vi "SmoothWaveform.vi"(0 "Waveform":waveform(dbl)={"t0"=timestamp(3461330237.7970004 s since 1904-01-01), "dt"=9.000000000000001e-07, "Y"=[]}, 1 "Smoothing Strength":T1=enum."20") -> (2 "Filtered data":waveform(dbl)={"t0"=timestamp(3461330237.7970004 s since 1904-01-01), "dt"=9.000000000000001e-07, "Y"=[]})   [LabVIEW 2010]
uses:
  FilterStrength.ctl
  <vilib>/Analysis/3filter.llb/Filter Passband Type.ctl
  <vilib>/Analysis/3filter.llb/Butterworth Filter (DBL).vi
  <vilib>/Analysis/NI_AALBase.lvlib
panel:
  in  "Draw Graph":bool
  out "XY Graph":cluster{dbl[], dbl[]}[](graph)
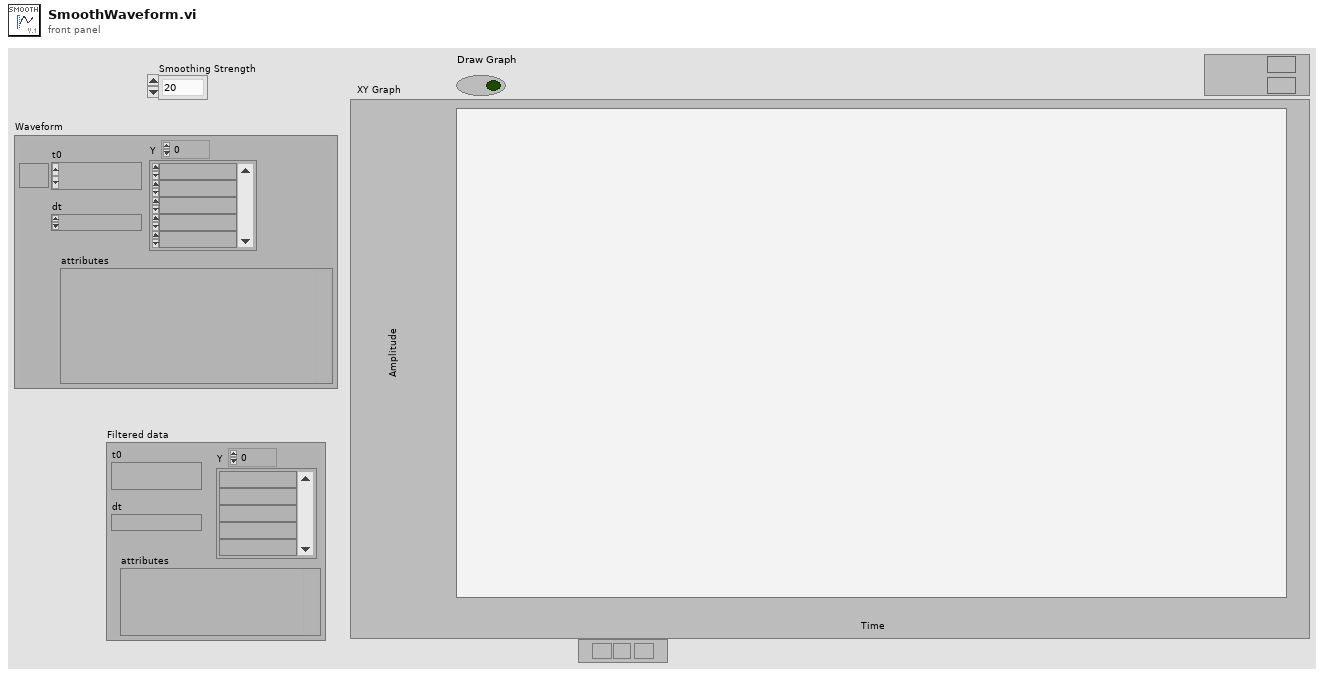
[diagram p1: front panel]
types:
  T1 = typedef "FilterStrength.ctl" = enum16{"Off", "10", "20", "50", "100", "200", "500", "1000"}
  T2 = typedef "NI_AALBase.lvlib/Filter Passband Type.ctl" = enum32{"Lowpass", "Highpass", "Bandpass", "Bandstop"}
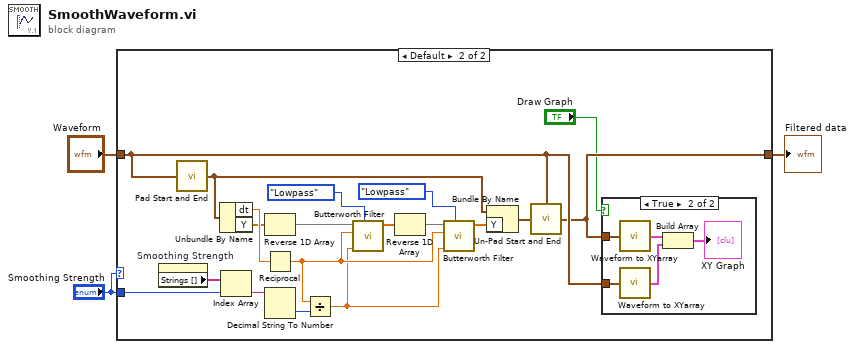
[diagram p0: block diagram]
diagram:
  n1 = case shown="Default" "Smoothing Strength" {
    tunnel: "Smoothing Strength" -> [_ w21]
    tunnel: "Waveform" -> [w4 w16]
    tunnel: [w4 w15] -> w2
    frame "Off" {
    }
    frame Default {
      n2 = property on="Smoothing Strength" class="Enum (strict)"() -> ("Strings []"=w22:string[])  [unwired: 2 in, 2 out]
      n3 = call "Pad Start and End.vi"("Waveform"=w16) -> ("Padded waveform"=w14:waveform(dbl))
      n4 = Unbundle By Name(w14) -> ("dt"=w18:dbl, "Y"=w17:dbl[])
      n5 = Index Array(array=w22, index=w21) -> (element=w20:string)
      n6 = Reverse 1D Array(array=w17) -> (reversed array=w12:dbl[])
      n7 = Reciprocal(x=w18) -> (1/x=w8:dbl)
      n8 = Decimal String To Number(string=w20) -> (number=w19:i32)  [unwired: 2 in, 1 out]
      n9 = Divide(x=w8, y=w19) -> (x/y=w7:dbl)
      n10 = call-poly <vilib>:"Butterworth Filter.vi"("filter type"=Filter_Passband_Type."Lowpass", "low cutoff freq: fl"=w7, "sampling freq: fs"=w8, "X"=w12) -> ("Filtered X"=w11:dbl[])  [unwired: 4 in, 1 out]
      n11 = Reverse 1D Array(array=w11) -> (reversed array=w9:dbl[])
      n12 = call-poly <vilib>:"Butterworth Filter.vi"("filter type"=Filter_Passband_Type."Lowpass", "low cutoff freq: fl"=w7, "sampling freq: fs"=w8, "X"=w9) -> ("Filtered X"=w6:dbl[])  [unwired: 4 in, 1 out]
      n13 = Bundle By Name(cluster=w14, "Y"=w6) -> (w13:waveform(dbl))
      n14 = call "Un-Pad Start and End.vi"("Padded Waveform"=w13, "Original Waveform"=w16) -> ("Un-padded Waveform"=w15:waveform(dbl))
      n15 = case shown="True" "Draw Graph" {
        tunnel: w16 -> [_ w28]
        tunnel: w15 -> [_ w27]
        frame False {
        }
        frame True {
          n16 = call "Waveform to XYarray.vi"("Waveform In"=w27) -> ("Single Plot"=w25:cluster{"X array":dbl[], "Y array":dbl[]})
          n17 = call "Waveform to XYarray.vi"("Waveform In"=w28) -> ("Single Plot"=w24:cluster{"X array":dbl[], "Y array":dbl[]})
          n18 = Build Array(w25, w24) -> (→"XY Graph":cluster{"X array":dbl[], "Y array":dbl[]}[])
        }
      }
    }
  }
  "Filtered data" <- w2
